vi "Configure Mask Test (Position).vi"(0 "VISA resource name":refnum<visa-resource-name>, 1 "Enable Bind (F: Disable)":bool, 5 "X1 (0.0002 S)":dbl=0.0002, 9 "X Delta (0.0004 S)":dbl=0.0004, 11 "error in (no error)":errorcluster, 12 "Y1 (-3 V)":dbl=-3.0, 13 "Y2 (3 V)":dbl=3.0) -> (4 "VISA resource name out":refnum<visa-resource-name>, 15 "error out":errorcluster)   [LabVIEW 2015, in "Agilent 2000 3000 X-Series.lvlib"]
doc: "Configure the position settings of mask test."
uses:
  <instrlib>/Agilent 2000 3000 X-Series/Agilent 2000 3000 X-Series.lvlib
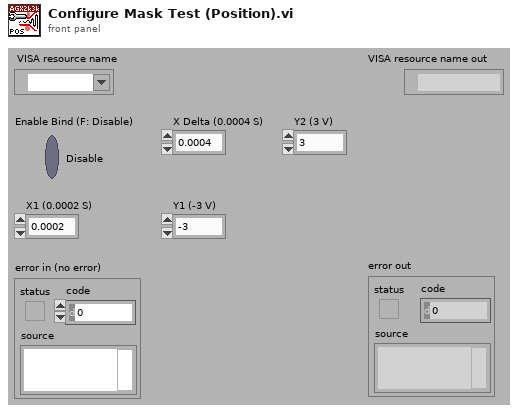
[diagram p1: front panel]
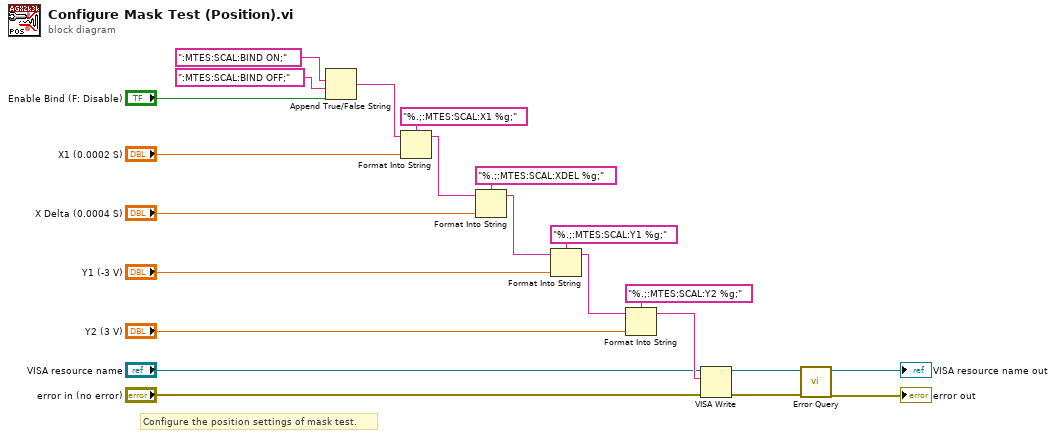
[diagram p0: block diagram]
diagram:
  # "Configure the position settings of mask test."
  n1 = Append True/False String(1:"Enable Bind (F: Disable)", 2:":MTES:SCAL:BIND OFF;", 3:":MTES:SCAL:BIND ON;") -> (0:w19:string)  [unwired: 1 out]
  n2 = Format Into String(format string="%.;:MTES:SCAL:X1 %g;", initial string=w19, "X1 (0.0002 S)") -> (resulting string=w16:string)  [unwired: 1 in, 1 out]
  n3 = Format Into String(format string="%.;:MTES:SCAL:XDEL %g;", initial string=w16, "X Delta (0.0004 S)") -> (resulting string=w13:string)  [unwired: 1 in, 1 out]
  n4 = Format Into String(format string="%.;:MTES:SCAL:Y1 %g;", initial string=w13, "Y1 (-3 V)") -> (resulting string=w10:string)  [unwired: 1 in, 1 out]
  n5 = Format Into String(format string="%.;:MTES:SCAL:Y2 %g;", initial string=w10, "Y2 (3 V)") -> (resulting string=w7:string)  [unwired: 1 in, 1 out]
  n6 = VISA Write(VISA resource name="VISA resource name", write buffer=w7, error in (no error)="error in (no error)") -> (VISA resource name out=w4:refnum<visa-resource-name>, error out=w3:errorcluster)  [unwired: 1 out]
  n7 = call <instrlib>:"Error Query.vi"("error in (no error)"=w3, "VISA resource name"=w4) -> ("error out"=→"error out":errorcluster, "VISA resource name out"=→"VISA resource name out":refnum<visa-resource-name>)  [unwired: 8 out]
